vi "Constants.vi"() -> ()   [LabVIEW 2015, in "UDP-Custom-Device Shared.lvlib"]
doc: "Use this Global VI to access the GUIDs assigned to the page resources of the Custom Device."
uses:
  UDP-Custom-Device Shared.lvlib
panel:
  in  "Tab Control":enum32{"GUIDS", "Constants", "Properties"}(tab)
  in  "Status Channel Page GUID":string="dbe1565a-647c-4128-a5fd-e9726cfe8b31"
  in  "Status Section Page GUID":string="4fe98813-0d2f-43b7-911c-1a5a6e2d5286"
  in  "Rx Channel Page GUID":string="8ede79f1-e06f-41dd-88ab-5074f11d4bb7"
  in  "Tx Section Page GUID":string="83990986-7c5f-4a4f-9521-e5ef95a941a7"
  in  "Rx Section Page GUID":string="e4cf9946-87d0-45cb-83bc-815ce28b6d77"
  in  "UDP-Custom-Device":string="1dbe19ca-57a1-40f3-b205-33efa5cbd18f"
  in  "Rx FIFO Timeout":string="Rx FIFO Timeout"
  in  "Rx FIFO Polling Rate":string="Rx FIFO Polling Rate"
  in  "Rx Channel Destination Ref":string="Rx Channel Destination Ref"
  in  "Rx Channel Description":string="Rx Channel Description"
  in  "Rx Channel Destination Path":string="Rx Channel Destination Path"
  in  "Tx Remove Channel Button ID":string="NIVS_UDPDataLink_Tx_RemoveChannels"
  in  "Tx Channel Delete Indices":string="Tx Channel Delete Indices"
  in  "Tx Channel Refs":string="Tx Channel Refs"
  in  "Tx Channel Paths":string="Tx Channel Paths"
  in  "Tx Channel Names":string="Tx Channel Names"
  in  "Export File Location":string="Export File Location"
  in  "Export to File Status":string="Export to File Status"
  in  "Decimation":string="Decimation"
  in  "IP of Local NIC State":string="IP of Local NIC State"
  in  "Auto-Assign IP":string="Auto-Assign IP"
  in  "TimeStamp Ref":string="TimeStamp Ref"
  in  "Server Port":string="Server Port"
  in  "IP of Remote NIC":string="IP of Remote NIC"
  in  "IP of Local NIC":string="IP of Local NIC"
  in  "Compiled.Settings":string="Compiled.Settings"
  in  "Rx Channel Delete Indices":string="Rx Channel Delete Indices"
  in  "Rx Channel Names":string="Rx Channel Names"
  in  "Rx Channel Paths":string="Rx Channel Paths"
  in  "Rx Channel Refs":string="Rx Channel Refs"
  # "Main Page Properties"
  # "Rx Section Properties"
  # "Tx Section Properties"
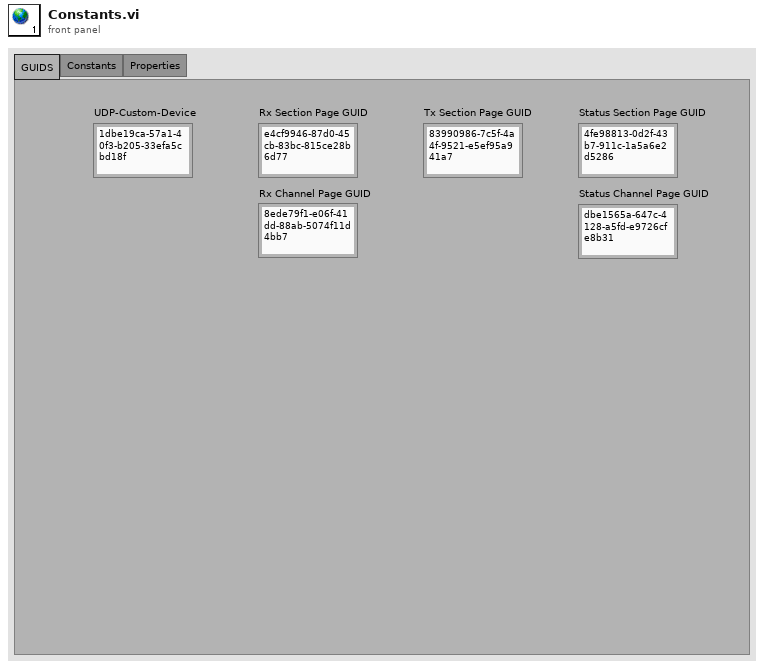
[diagram p1: front panel]
diagram:
